vi "WPI_DigitalOutputIsPulsing.vi"(8 "error in (no error)":errorcluster, 11 "DigitalOutputDevRef":T1={"DIO Channel"=enum."DIO 1", "DevStatus"={"status"=FALSE, "code"=0, "source"=""}}) -> (0 "error out":errorcluster, 2 "IsPulsing?":bool, 3 "DigitalOutputDevRef":T1={"DIO Channel"=enum."DIO 1", "DevStatus"={"status"=FALSE, "code"=0, "source"=""}})   [LabVIEW 2017]
doc: "Returns whether the digital output is emitting a pulse.\n\nThis software is licensed. Open the labview\\readme\\WPI Robotics Library Open Source License.txt file for more information."
uses:
  <vilib>/Rock Robotics/WPI/DigitalOutput/WPI_DigitalOutputDevRef.ctl
  <vilib>/Rock Robotics/SystemInterfaces/DIO/FPGA_DIOChannel.ctl
  <vilib>/Rock Robotics/WPI/DigitalModule/WPI_DigitalModuleDIOCacheOp.ctl
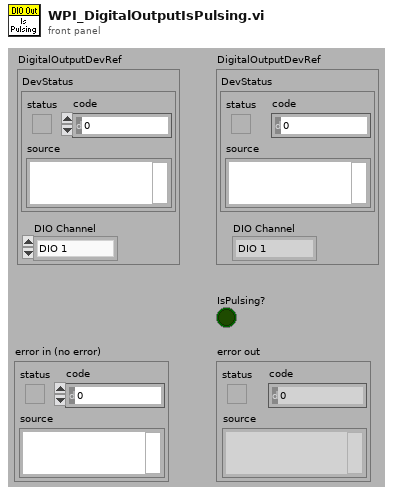
[diagram p1: front panel]
types:
  T1 = typedef "WPI_DigitalOutputDevRef.ctl" = cluster{"DIO Channel":T2, "DevStatus":errorcluster}
  T2 = typedef "FPGA_DIOChannel.ctl" = enum8{"DIO 0", "DIO 1", "DIO 2", "DIO 3", "DIO 4", "DIO 5", "DIO 6", "DIO 7", "DIO 8", "DIO 9", "DIO MXP 0", "DIO MXP 1", "DIO MXP 2", "DIO MXP 3", "DIO MXP 4", "DIO MXP 5", "DIO MXP 6", "DIO MXP 7", "DIO MXP 8", "DIO MXP 9", "DIO MXP 10", "DIO MXP 11", "DIO MXP 12", "DIO MXP 13", "DIO MXP 14", "DIO MXP 15", "SPI Port CS1", "SPI Port CS2", "SPI Port CS3", "SPI Port MISO", "SPI Port MOSI", "Invalid"}
  T3 = typedef "WPI_DigitalModuleDIOCacheOp.ctl" = enum16{"Acquire", "Release", "Status"}
  T4 = typedef "WPI_DigitalModuleDeviceRef.ctl" = cluster{"DevStatus":errorcluster}
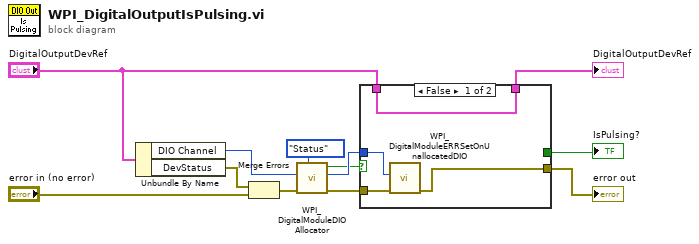
[diagram p0: block diagram]
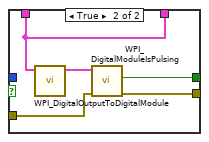
[diagram p2: hidden frame]
diagram:
  n1 = Unbundle By Name("DigitalOutputDevRef") -> ("DIO Channel"=w8:T2, "DevStatus"=w4:errorcluster)
  n2 = Merge Errors(w4, "error in (no error)") -> (w3:errorcluster)
  n3 = call <vilib>:"WPI_DigitalModuleDIOAllocator.vi"("AllocatedDIOMutex"=WPI_DigitalModuleDIOCacheOp."Status", "error in (no error)"=w3, "DIOChannel"=w8) -> ("error out"=w5:errorcluster, "Allocated DIOChannel"=w7:T2, "AllocatedDIO"=w6:bool)  [unwired: 1 in, 5 out]
  n4 = case shown="False" w6 {
    tunnel: [w15 w19] -> w1
    tunnel: w7 -> [w14 _]
    tunnel: "DigitalOutputDevRef" -> [w13 w17]
    tunnel: w5 -> [w16 w20]
    tunnel: [_ w18] -> w10
    tunnel: [w13 w17] -> w2
    frame False {
      n5 = call <vilib>:"WPI_DigitalModuleERRSetOnUnallocatedDIO.vi"("error in (no error)"=w16, "DIOChannel"=w14) -> ("error out"=w15:errorcluster)  [unwired: 9 in]
    }
    frame True {
      n6 = call <vilib>:"WPI_DigitalOutputToDigitalModule.vi"("DigitalOutputDevRef"=w17) -> ("DigitalModuleDevRef"=w21:T4)  [unwired: 10 out]
      n7 = call <vilib>:"WPI_DigitalModuleIsPulsing.vi"("error in (no error)"=w20, "DigitalModuleDevRef"=w21) -> ("error out"=w19:errorcluster, "IsPulsing?"=w18:bool)  [unwired: 1 in, 7 out]
    }
  }
  "DigitalOutputDevRef" <- w2
  "error out" <- w1
  "IsPulsing?" <- w10
